vi "INI read instruments.vi"(8 "error in (no error)":T2) -> (0 "error out":T2, 2 "Timing module":tag, 3 "mmWave instr":T1={"TX_DAC"="Rx_ADC", "TX_FPGA"="RX_FPGA", "IF"="IF_mod", "RX_ADC"="Rx_ADC", "RX_FPGA"="RX_FPGA"} caption="data")   [LabVIEW 2019, in "Shared.lvlib"]
uses:
  Shared.lvlib
  mmWave HW Control/HW TXRX resources cluster.ctl
  System GV.vi
  <vilib>/Utility/error.llb/Error Cluster From Error Code.vi
  <vilib>/ErrorRing/Error Ring.xnode
  <vilib>/Utility/config.llb/NI_LVConfig.lvlib
  mmWave HW Control/mmWave HW Control.lvlib
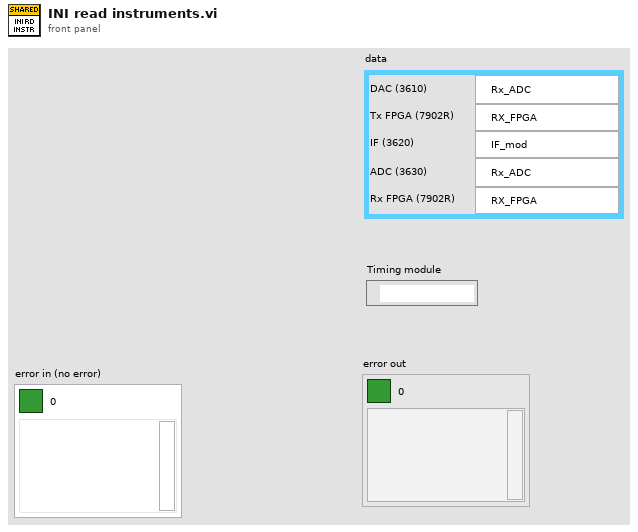
[diagram p1: front panel]
types:
  T1 = typedef "mmWave HW Control.lvlib/HW TXRX resources cluster.ctl" = cluster{"TX_DAC":refnum<visa-resource-name>, "TX_FPGA":tag, "IF":tag, "RX_ADC":refnum<visa-resource-name>, "RX_FPGA":tag}
  T2 = cluster{"Boolean Round":bool, "code":i32, "source":string}
  T3 = cluster{"TX_DAC":string, "TX_FPGA":string, "IF":string, "RX_ADC":string, "RX_FPGA":string}
  T4 = typedef "NI_LVConfig.lvlib/Config Data RefNum.ctl" = refnum<k1>
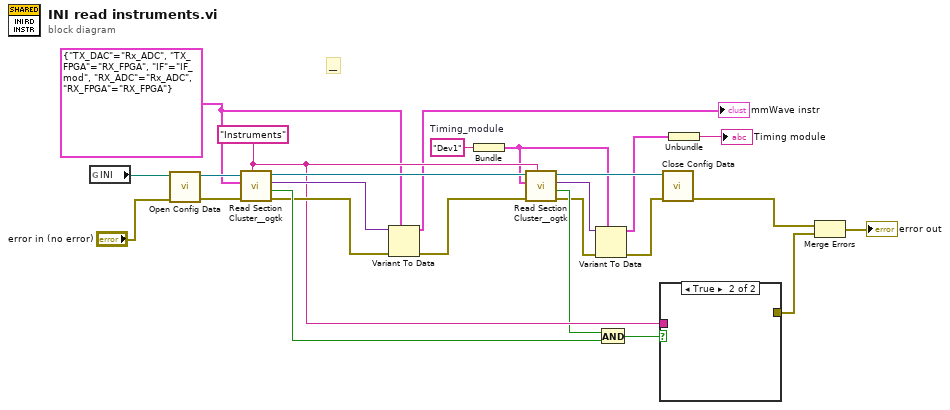
[diagram p0: block diagram]
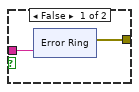
[diagram p2: hidden frame]
diagram:
  w19 = "Dev1"  # Timing_module
  w2 = T3 {"TX_DAC"="Rx_ADC", "TX_FPGA"="RX_FPGA", "IF"="IF_mod", "RX_ADC"="Rx_ADC", "RX_FPGA"="RX_FPGA"} ("HW.RX resources")
  w17 = "Instruments" ("section (optional)")
  # "__"
  n1 = global read "System GV.vi" "INI"() -> (w23:path)
  n2 = call <vilib>:"Open Config Data.vi"("error in (no error)"="error in (no error)", "configuration file path"=w23) -> ("error out"=w24:errorcluster, "refnum"=w25:T4)  [unwired: 7 in, 1 out]
  n3 = call <userlib>:"Read Section Cluster__ogtk.vi"("section (optional)"=w17, "error in (no error)"=w24, "Section Formatted Cluster Type"=w2, "refnum"=w25) -> ("error out"=w20:errorcluster, "all found?"=w22:bool, "Section Formatted Cluster"=w21:variant, "dup refnum"=w18:T4)  [unwired: 3 in, 1 out]
  n4 = Variant To Data(error in=w20, type=w2, Variant=w21) -> (data=→"mmWave instr":T3, error out=w15:errorcluster)
  n5 = Bundle("Timing_module"=w19) -> (w6:cluster{"Timing_module":string})  [unwired: 1 in]
  n6 = call <userlib>:"Read Section Cluster__ogtk.vi"("section (optional)"=w17, "error in (no error)"=w15, "Section Formatted Cluster Type"=w6, "refnum"=w18) -> ("error out"=w12:errorcluster, "all found?"=w13:bool, "Section Formatted Cluster"=w10:variant, "dup refnum"=w16:T4)  [unwired: 3 in, 1 out]
  n7 = Variant To Data(error in=w12, type=w6, Variant=w10) -> (data=w7:cluster{"Timing_module":string}, error out=w11:errorcluster)
  n8 = And(x=w13, y=w22) -> (x .and. y?=w14:bool)
  n9 = case shown="True" w14 {
    tunnel: w17 -> [w27 _]
    tunnel: [w26 _] -> w4
    frame False {
      n10 = xnode "Error Ring"("parameter 0"=w27) -> ("error out"=w26:errorcluster)
    }
    frame True {
    }
  }
  n11 = call <vilib>:"Close Config Data.vi"("error in (no error)"=w11, "refnum"=w16) -> ("error out"=w5:errorcluster)  [unwired: 8 in, 1 out]
  n12 = Unbundle(w7) -> ("Timing_module"=→"Timing module":string)
  n13 = Merge Errors(w5, w4) -> (→"error out":errorcluster)
